vi "Get Feature Colour.vi"(11 "Feature Type":u16) -> (3 "color":u32)   [LabVIEW 2024]
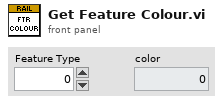
[diagram p1: front panel]
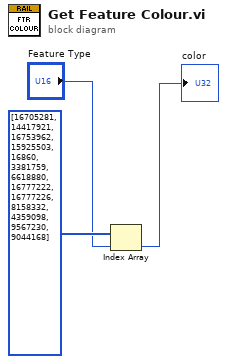
[diagram p0: block diagram]
diagram:
  n1 = Index Array(array=u32[] [16705281, 14417921, 16753962, 15925503, 16860, 3381759, 6618880, 16777222, 16777226, 8158332, 4359098, 9567230, 9044168], index="Feature Type") -> (element=→"color":u32)
